vi "Controller Configuration Loop.vi"(7 "Sync Objects":T1, 8 "error in (no error)":errorcluster, 11 "FOFB Configuration":T5={"FOFB Parameters"={"Network"={"FOFB Controller IP"="", "LNLS Control Network IP"="", "LNLS Control Network Power Supplies TCP Port"=0, "LNLS Control Network FOFB Configuration TCP Port"=0, "Data Server TCP Port"=0, "Monitoring Data TCP Port"=0, "Configuration GUI TCP Port"=0, "TCP Listening Timeout"=0}, "Fast Acquisition"={"Acquisition Period"=0, "Data Buffer Size"=0}, "Response Matrix Measurement"={"Step Amplitude"=0.0, "Time Between Steps"=0, "Step Duration"=0, "Number of Averages"=0}, "Correction Algorithm"={"Correction Period"=0, "Reference Orbit Path"=path "", "Response Matrix Path"=path "", "Correction Matrix Path"=path "", "Horizontal Correction Factor"=0.0, "Vertical Correction Factor"=0.0, "Beam Current FOFB Threshold"=0.0, "Decouple H-V"=FALSE}, "Acquisition Network"=[], "Actuation Network"=[]}, "Number of Acquisition Chassis"=0, "Number of Actuation Chassis"=0, "Number of BPM Readings"=0, "BPM Reading Names"=[], "Selected BPM Readings"=[0, 1, 2, 3, 4, 5, 6, 7, 8, 9, 10, 11, 12, 13, 14, 15, 16, 17, 18, 19, 20, 21, 22, 23, 24, 25, 26, 27, 28, 29, 30, 31, 32, 33, 34, 35, 36, 37, 38, 39, 40, 41, 42, 43, 44, 45, 46, 47, 48, 49], "Number of Correctors"=0, "Corrector Names"=[], "Selected Correctors"=[0, 1, 2, 3, 4, 5, 6, 7, 8, 9, 10, 11, 12, 13, 14, 15, 16, 17, 18, 19, 20, 21, 22, 23, 24, 25, 26, 27, 28, 29, 30, 31, 32, 33, 34, 35, 36, 37, 38, 39, 40, 41, 42, 43, 44, 45, 46, 47, 48, 49], "Reference Orbit"=[], "Response Matrix"=[], "Correction Matrix"=[], "Acquisition Chassis Names"=[], "Actuation Chassis Names"=[], "Acquisition Variables"=[], "Actuation Variables"=[], "PS Matrix Mapping"=[], "Inverse PS Matrix Mapping"=[], "Response Matrix Beam Energy (MeV)"=0.0, "PID Parameters"=[], "BPM Planes"=[], "Corrector Planes"=[], "RMM Step Factor"=[]}) -> (0 "error out":errorcluster)   [LabVIEW 2011, in "Controller VIs.lvlib"]
uses:
  Controller VIs.lvlib
  Types Definitions/Type FOFB Configuration.ctl
  Types Definitions/Type FOFB Parameters.ctl
  Types Definitions/Type Network Configuration.ctl
  Types Definitions/Type FA Configuration.ctl
  Types Definitions/Type Response Matrix Measurement Configuration.ctl
  Types Definitions/Type Correction Algorithm Configuration.ctl
  Types Definitions/Type Acquisition Network Configuration.ctl
  Types Definitions/Type Actuation Network Configuration.ctl
  Types Definitions/Type PID Parameters.ctl
  Types Definitions/Type Synchronization Objects.ctl
  Types Definitions/Type Blocking Synchronization Objects.ctl
  Types Definitions/Type FA Request Parameters.ctl
  Types Definitions/Type BPM and PS select cluster.ctl
  Types Definitions/Type FA File Parameters.ctl
  Types Definitions/Type Monitoring Data.ctl
  Types Definitions/Type Diagnostics Data.ctl
  Types Definitions/Type CPU Loads Array.ctl
  Types Definitions/Type CPU Loads.ctl
  Types Definitions/Type Non-blocking Synchronization Objects.ctl
  Types Definitions/Type FOFB Variables.ctl
  Types Definitions/Type Actuation State.ctl
  <vilib>/Platform/TimedLoop/XDataNode/timing_clust.ctl
  <vilib>/Platform/TimedLoop/XDataNode/nitl_modes.ctl
  <vilib>/Platform/TimedLoop/XDataNode/wakeup.ctl
  Types Definitions/Type Configuration Data (GUI to Controller).ctl
  <vilib>/rtutility.llb/RT Debug String.vi
  <vilib>/Platform/TimedLoop/XDataNode/XDataNode.xnode
  Type Definitions.lvlib
  Log VIs.lvlib
  Misc VIs.lvlib
  <vilib>/Platform/TimedLoop/XDataNode/XDNodeRunTimeDep.lvlib
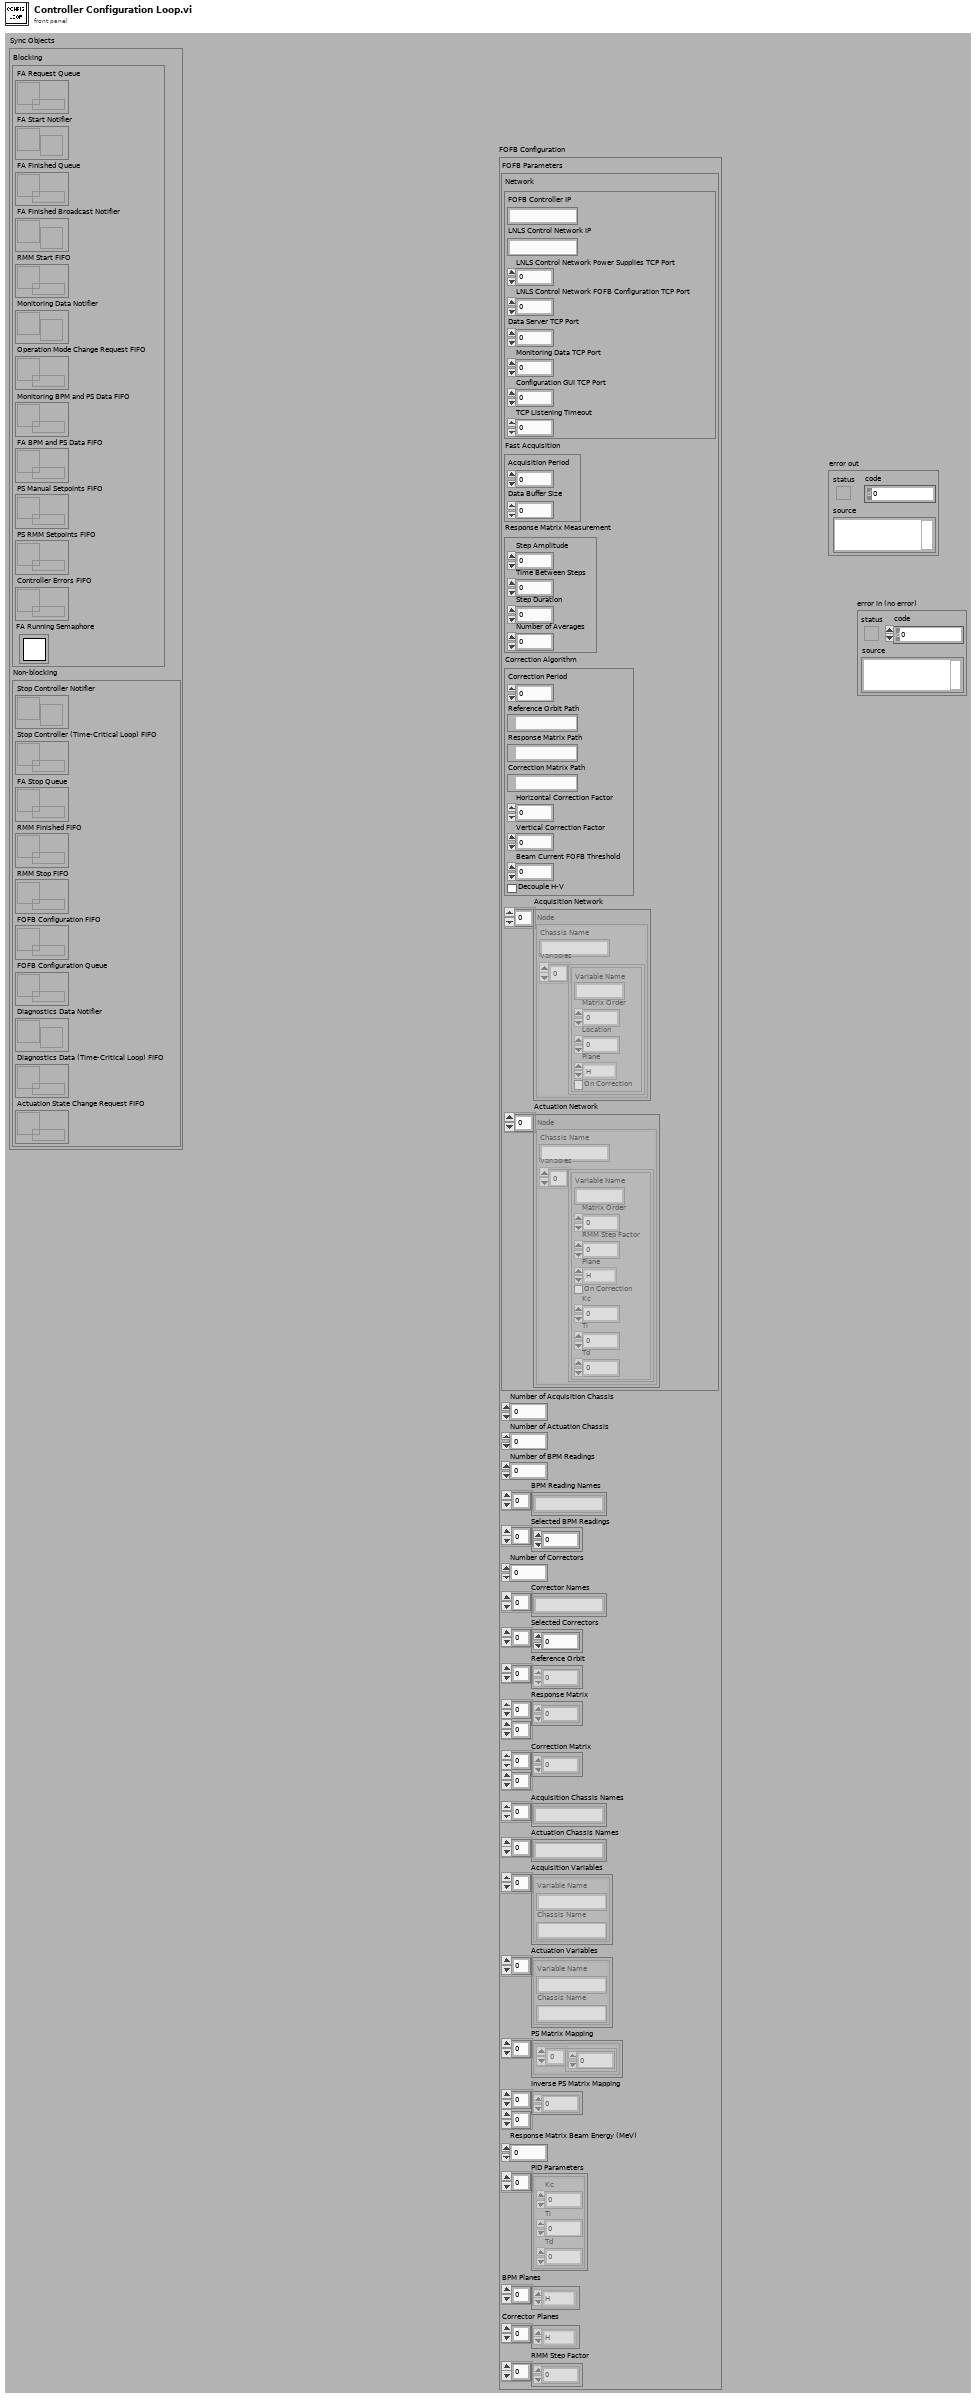
[diagram p1: front panel]
types:
  T1 = typedef "Type Definitions.lvlib/Type Synchronization Objects.ctl" = cluster{"Blocking":T2, "Non-blocking":T4}
  T2 = typedef "Type Definitions.lvlib/Type Blocking Synchronization Objects.ctl" = cluster{"FA Request Queue":refnum<queue>, "FA Start Notifier":refnum<notifier>, "FA Finished Queue":refnum<queue>, "FA Finished Broadcast Notifier":refnum<notifier>, "RMM Start FIFO":refnum<k33>, "Monitoring Data Notifier":refnum<notifier>, "Operation Mode Change Request FIFO":refnum<k33>, "Monitoring BPM and PS Data FIFO":refnum<k33>, "FA BPM and PS Data FIFO":refnum<k33>, "PS Manual Setpoints FIFO":refnum<k33>, "PS RMM Setpoints FIFO":refnum<k33>, "Controller Errors FIFO":refnum<k33>, "FA Running Semaphore":T3}
  T3 = typedef "Semaphore RefNum" = refnum<k1>
  T4 = typedef "Type Definitions.lvlib/Type Non-blocking Synchronization Objects.ctl" = cluster{"Stop Controller Notifier":refnum<notifier>, "Stop Controller (Time-Critical Loop) FIFO":refnum<k33>, "FA Stop Queue":refnum<queue>, "RMM Finished FIFO":refnum<k33>, "RMM Stop FIFO":refnum<k33>, "FOFB Configuration FIFO":refnum<k33>, "FOFB Configuration Queue":refnum<queue>, "Diagnostics Data Notifier":refnum<notifier>, "Diagnostics Data (Time-Critical Loop) FIFO":refnum<k33>, "Actuation State Change Request FIFO":refnum<k33>}
  T5 = typedef "Type Definitions.lvlib/Type FOFB Configuration.ctl" = cluster{"FOFB Parameters":T6, "Number of Acquisition Chassis":i32, "Number of Actuation Chassis":i32, "Number of BPM Readings":i32, "BPM Reading Names":string[], "Selected BPM Readings":u32[], "Number of Correctors":i32, "Corrector Names":string[], "Selected Correctors":u32[], "Reference Orbit":dbl[], "Response Matrix":dbl[][], "Correction Matrix":dbl[][], "Acquisition Chassis Names":string[], "Actuation Chassis Names":string[], "Acquisition Variables":cluster{"Variable Name":string, "Chassis Name":string}[], "Actuation Variables":cluster{"Variable Name":string, "Chassis Name":string}[], "PS Matrix Mapping":cluster{u32[]}[], "Inverse PS Matrix Mapping":u32[][], "Response Matrix Beam Energy (MeV)":dbl, "PID Parameters":T13[], "BPM Planes":enum8{"H", "V"}[], "Corrector Planes":enum8{"H", "V"}[], "RMM Step Factor":dbl[]}
  T6 = typedef "Type Definitions.lvlib/Type FOFB Parameters.ctl" = cluster{"Network":T7, "Fast Acquisition":T8, "Response Matrix Measurement":T9, "Correction Algorithm":T10, "Acquisition Network":T11, "Actuation Network":T12}
  T7 = typedef "Type Definitions.lvlib/Type Network Configuration.ctl" = cluster{"FOFB Controller IP":string, "LNLS Control Network IP":string, "LNLS Control Network Power Supplies TCP Port":u16, "LNLS Control Network FOFB Configuration TCP Port":u16, "Data Server TCP Port":u16, "Monitoring Data TCP Port":u16, "Configuration GUI TCP Port":u16, "TCP Listening Timeout":i32}
  T8 = typedef "Type Definitions.lvlib/Type FA Configuration.ctl" = cluster{"Acquisition Period":u32, "Data Buffer Size":u32}
  T9 = typedef "Type Definitions.lvlib/Type Response Matrix Measurement Configuration.ctl" = cluster{"Step Amplitude":dbl, "Time Between Steps":u32, "Step Duration":u32, "Number of Averages":u32}
  T10 = typedef "Type Definitions.lvlib/Type Correction Algorithm Configuration.ctl" = cluster{"Correction Period":u32, "Reference Orbit Path":path, "Response Matrix Path":path, "Correction Matrix Path":path, "Horizontal Correction Factor":dbl, "Vertical Correction Factor":dbl, "Beam Current FOFB Threshold":dbl, "Decouple H-V":bool}
  T11 = typedef "Type Definitions.lvlib/Type Acquisition Network Configuration.ctl" = cluster{"Chassis Name":string, "Variables":cluster{"Variable Name":string, "Matrix Order":u32, "Location":dbl, "Plane":enum8{"H", "V"}, "On Correction":bool}[]}[]
  T12 = typedef "Type Definitions.lvlib/Type Actuation Network Configuration.ctl" = cluster{"Chassis Name":string, "Variables":cluster{"Variable Name":string, "Matrix Order":u32, "RMM Step Factor":dbl, "Plane":enum8{"H", "V"}, "On Correction":bool, "Kc":dbl, "Ti":dbl, "Td":dbl}[]}[]
  T13 = typedef "Type Definitions.lvlib/Type PID Parameters.ctl" = cluster{"Kc":fxp<+/-,16,8>, "Ti":fxp<+/-,16,8>, "Td":fxp<+/-,16,8>}
  T14 = enum16{"Idle", "Wait Connection", "Read Data", "Process Data", "Write Data", "Close Connection"}
  T15 = typedef "XDNodeRunTimeDep.lvlib/timing_clust.ctl" = cluster{"Expected End [f-1]":u64, "Actual End [f-1]":u64, "Finished Late? [f-1]":bool, "Expected End [i-1]":u64, "Actual End [i-1]":u64, "Finished Late? [i-1]":bool, "Expected Start [i]":u64, "Actual Start [i]":u64, "Expected Start [f]":u64, "Actual Start [f]":u64, "Source Name":string, "Structure Name":string, "Period":i64, "Deadline":i64, "Offset":i64, "Start":i64, "Priority":i32, "Timeout":i32, "Mode":T16, "Wakeup Reason":T17, "Error":errorcluster, "Source Type":string, "Secondary Source Type":string, "Global End Time":u64, "Global Start Time":u64, "Frame Duration":u64, "Iteration Duration":u64, "Assigned CPU":i32, "I/O Scan Engine Mode":u32}
  T16 = typedef "XDNodeRunTimeDep.lvlib/nitl_modes.ctl" = enum32{"No Change", "Process missed periods, maintain original phase", "Discard missed periods, maintain original phase", "Process missed periods, ignore original phase", "Discard missed periods, ignore original phase"}
  T17 = typedef "XDNodeRunTimeDep.lvlib/wakeup.ctl" = enum32{"Normal", "Aborted", "Asynchronous wakeup", "Timing source error", "Timed loop error", "Timeout"}
  T18 = typedef "Type Definitions.lvlib/Type Configuration Data (GUI to Controller).ctl" = cluster{"Operation Mode":enum16{"Idle Mode", "Error Mode", "Manual Mode", "FOFB Mode", "RMM Mode"}[], "Update Controller Soft Configuration":bool[], "Trigger RT Execution Trace":string[]}
  T19 = typedef "Type Definitions.lvlib/Type Configuration Change Acknowledge (Controller to GUI).ctl" = cluster{"Operation Mode ACK":bool[]}
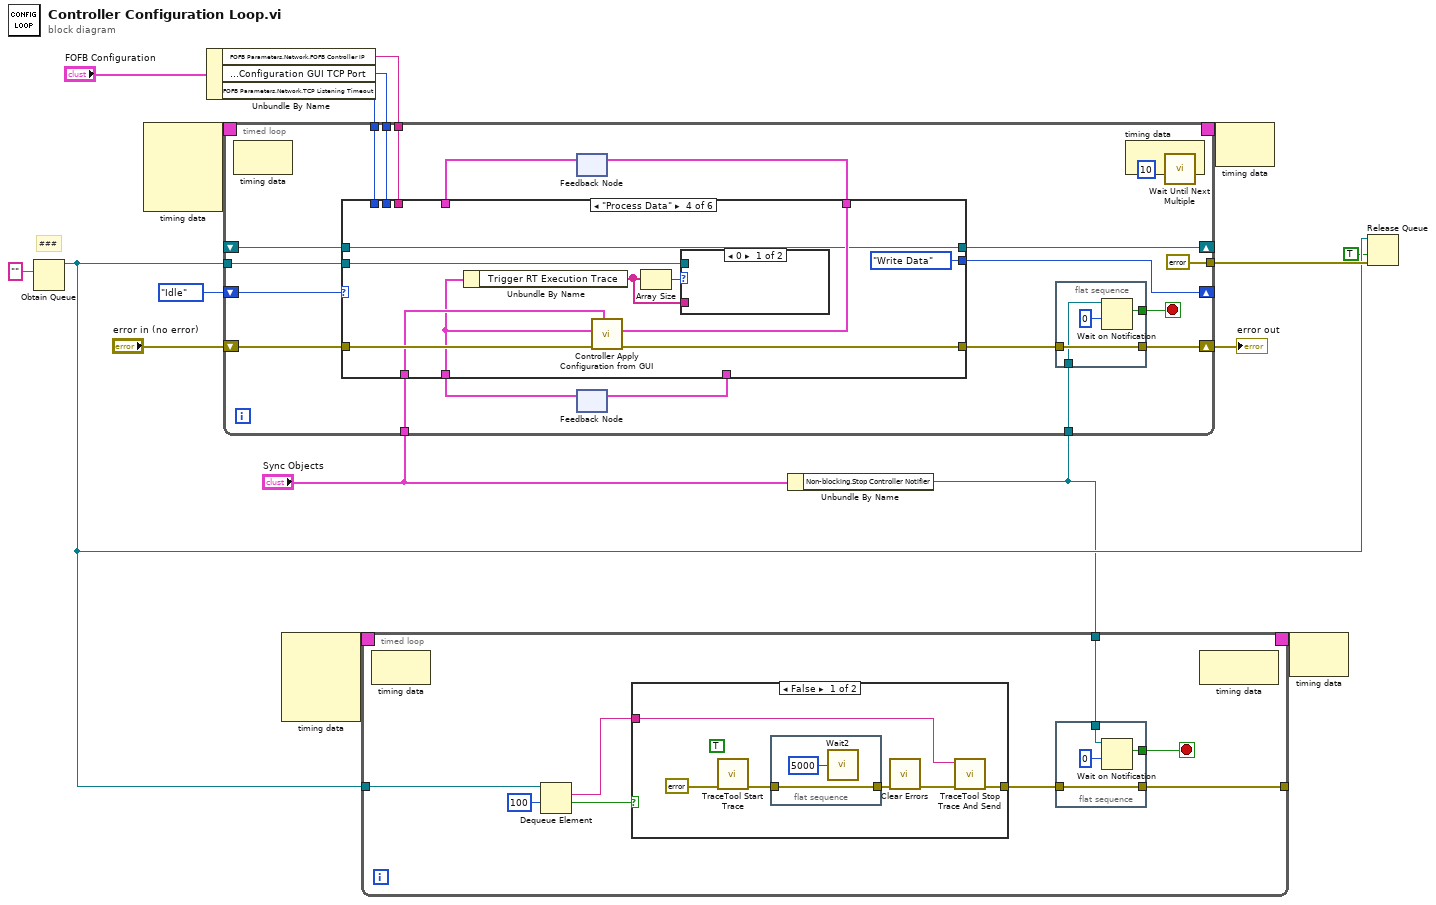
[diagram p0: block diagram]
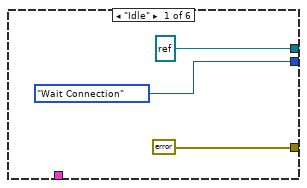
[diagram p3: hidden frame]
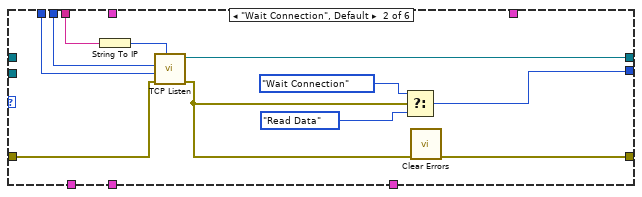
[diagram p4: hidden frame]
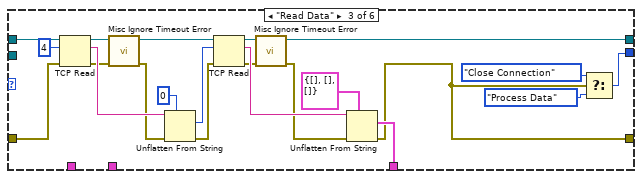
[diagram p5: hidden frame]
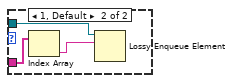
[diagram p6: hidden frame]
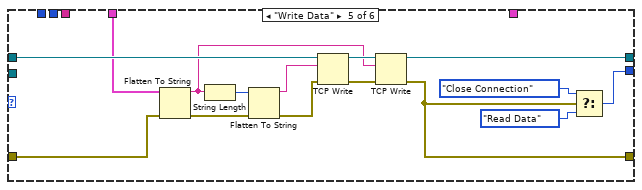
[diagram p7: hidden frame]
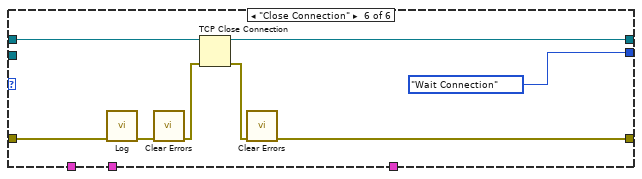
[diagram p8: hidden frame]
diagram:
  # "###"
  n1 = Obtain Queue(element data type="" ("Host IP Address")) -> (queue out=w3:refnum<queue>)  [unwired: 4 in, 2 out]
  n2 = node-c288() -> (w9:T15)  [unwired: 4 in]
  n3 = Unbundle By Name("FOFB Configuration") -> ("FOFB Parameters.Network.FOFB Controller IP"=w16:string, "FOFB Parameters.Network.Configuration GUI TCP Port"=w10:u16, "FOFB Parameters.Network.TCP Listening Timeout"=w15:i32)
  n4 = node-c288() -> (w7:T15)  [unwired: 4 in]
  n5 = Unbundle By Name("Sync Objects") -> ("Non-blocking.Stop Controller Notifier"=w1:refnum<notifier>)
  n6 = timed-loop {
    tunnel: w16 -> [w37]
    tunnel: w10 -> [w36]
    tunnel: w15 -> [w35]
    shift-right: [w23] -> w13
    shift-left: "error in (no error)" -> [w32]
    shift-right: [w30] -> _
    shift-left: T14."Idle" ("f") -> [w31]
    shift-right: [w33] -> _
    shift-left: _ -> [w34]
    tunnel: w1 -> [w22]
    tunnel: "Sync Objects" -> [w27]
    timing: w9 -> [_]
    timing-out: [_] -> w8
    tunnel: w3 -> [w19]
    tunnel: [errorcluster {"status"=FALSE, "code"=0, "source"=""} ("error out")] -> w4
    stop <- w21 stop-if-true
    # "ms"
    n7 = node-c288() -> ()  [unwired: 1 in, 1 out]
    n8 = feedback #1() -> (w26:T19)  [unwired: 1 in]
    n9 = feedback #2() -> (w28:T18)  [unwired: 1 in]
    n10 = case shown="\"Process Data\"" w31 {
      tunnel: [refnum<k5> refnum ("connection ID") w57 w70 w84 w105 w113] -> w33
      tunnel: [T14."Wait Connection" ("f") w56 w66 T14."Write Data" ("f") w104 T14."Wait Connection" ("f")] -> w30
      tunnel: [errorcluster {"status"=FALSE, "code"=0, "source"=""} ("error out") w54 w58 w86 w103 w112] -> w24
      tunnel: w32 -> [_ w53 w69 w87 w93 w107]
      tunnel: w34 -> [_ _ w71 w84 w101 w106]
      tunnel: w37 -> [_ w52 _ _ _ _]
      tunnel: w36 -> [_ w50 _ _ _ _]
      tunnel: w35 -> [_ w49 _ _ _ _]
      tunnel: [_ _ w63 _ _ _] -> w29
      tunnel: w28 -> [_ _ _ w81 _ _]
      tunnel: w27 -> [_ _ _ w82 _ _]
      tunnel: w26 -> [_ _ _ _ w94 _]
      tunnel: [_ _ _ w85 _ _] -> w25
      tunnel: w19 -> [_ _ _ w78 _ _]
      frame "Idle" {
      }
      frame "Wait Connection", Default {
        n11 = String To IP(1:w52) -> (0:w51:u32)
        n12 = call <vilib>:"TCP Listen.vi"("net address"=w51, "error in (no error)"=w53, "timeout ms (wait forever: -1)"=w49, "port"=w50) -> ("error out"=w55:errorcluster, "connection ID"=w57:refnum<k5>)  [unwired: 3 in, 3 out]
        n13 = Select(t=T14."Wait Connection" ("f"), s=w55, f=T14."Read Data") -> (s? t:f=w56:T14)
        n14 = call <vilib>:"Clear Errors.vi"("error in (no error)"=w55) -> ("error out"=w54:errorcluster)  [unwired: 6 out]
      }
      frame "Read Data" {
        n15 = TCP Read(connection ID=w71, bytes to read=4, error in (no error)=w69) -> (connection ID out=w77:refnum<k5>, data out=w75:string, error out=w64:errorcluster)  [unwired: 2 in]
        n16 = call "Misc Ignore Timeout Error.vi"("error in (no error)"=w64) -> ("error out"=w62:errorcluster)  [unwired: 10 in]
        n17 = Unflatten From String(type=0 ("bytes to read"), binary string=w75, error in (no error)=w62) -> (value=w73:i32, error out=w61:errorcluster)  [unwired: 2 in, 1 out]
        n18 = TCP Read(connection ID=w77, bytes to read=w73, error in (no error)=w61) -> (connection ID out=w70:refnum<k5>, data out=w72:string, error out=w60:errorcluster)  [unwired: 2 in]
        n19 = call "Misc Ignore Timeout Error.vi"("error in (no error)"=w60) -> ("error out"=w59:errorcluster)  [unwired: 10 in]
        n20 = Unflatten From String(type=T18 {"Operation Mode"=[], "Update Controller Soft Configuration"=[], "Trigger RT Execution Trace"=[]} ("Configuration Data (GUI to Controller)"), binary string=w72, error in (no error)=w59) -> (value=w63:T18, error out=w58:errorcluster)  [unwired: 2 in, 1 out]
        n21 = Select(t=T14."Close Connection" ("f"), s=w58, f=T14."Process Data") -> (s? t:f=w66:T14)
      }
      frame "Process Data" {
        n22 = Unbundle By Name(w81) -> ("Trigger RT Execution Trace"=w79:string[])
        n23 = call "Controller Apply Configuration from GUI.vi"("Sync Objects"=w82, "error in (no error)"=w87, "Configuration Data (GUI to Controller)"=w81) -> ("error out"=w86:errorcluster, "Configuration Change Acknowledge (Controller to GUI)"=w85:T19)  [unwired: 7 in]
        n24 = Array Size(array=w79) -> (size(s)=w80:i32)
        n25 = case shown="0" w80 {
          tunnel: w79 -> [_ w90]
          tunnel: w78 -> [_ w88]
          frame 0 {
          }
          frame 1, Default {
            n26 = Index Array(array=w90) -> (element=w89:string)  [unwired: 1 in]
            n27 = Lossy Enqueue Element(queue=w88, element=w89) -> ()  [unwired: 1 in, 4 out]
          }
        }
      }
      frame "Write Data" {
        n28 = Flatten To String(anything=w94, error in (no error)=w93) -> (data string=w97:string, error out=w92:errorcluster)  [unwired: 2 in, 1 out]
        n29 = String Length(string=w97) -> (length=w99:i32)
        n30 = Flatten To String(anything=w99, error in (no error)=w92) -> (data string=w98:string, error out=w91:errorcluster)  [unwired: 2 in, 1 out]
        n31 = TCP Write(connection ID=w101, data in=w98, error in (no error)=w91) -> (connection ID out=w102:refnum<k5>, error out=w100:errorcluster)  [unwired: 2 out]
        n32 = TCP Write(connection ID=w102, data in=w97, error in (no error)=w100) -> (connection ID out=w105:refnum<k5>, error out=w103:errorcluster)  [unwired: 2 out]
        n33 = Select(t=T14."Close Connection" ("f"), s=w103, f=T14."Read Data") -> (s? t:f=w104:T14)
      }
      frame "Close Connection" {
        n34 = call "Log.vi"("error in (no error)"=w107) -> ("error out"=w110:errorcluster)  [unwired: 9 in, 1 out]
        n35 = call <vilib>:"Clear Errors.vi"("error in (no error)"=w110) -> ("error out"=w111:errorcluster)  [unwired: 6 in]
        n36 = TCP Close Connection(connection ID=w106, error in (no error)=w111) -> (connection ID out=w113:refnum<k5>, error out=w109:errorcluster)  [unwired: 1 in]
        n37 = call <vilib>:"Clear Errors.vi"("error in (no error)"=w109) -> ("error out"=w112:errorcluster)  [unwired: 6 in]
      }
    }
    n38 = feedback-in #1(w25) -> ()
    n39 = feedback-in #2(w29) -> ()
    n40 = flat-sequence {
      tunnel: [w42] -> w21
      tunnel: w24 -> [w41]
      tunnel: [w41] -> w23
      tunnel: w22 -> [w40]
      frame #0 {
        n41 = Wait on Notification(notifier=w40, timeout in ms (-1)=0) -> (notification=w42:bool)  [unwired: 2 in, 3 out]
      }
    }
    n42 = node-c288() -> ()  [unwired: 1 in, 1 out]
    n43 = call "Wait Until Next Multiple"("Count(mSec)"=u32 10) -> ()  [unwired: 1 out]
  }
  "error out" <- w13
  n44 = timed-loop {
    timing: w7 -> [_]
    timing-out: [_] -> w6
    tunnel: w3 -> [w119]
    tunnel: [w117] -> _
    tunnel: w1 -> [w116]
    stop <- w114 stop-if-true
    n45 = node-c288() -> ()  [unwired: 1 in, 1 out]
    n46 = Dequeue Element(queue=w119, timeout in ms (-1)=100) -> (element=w115:string, timed out?=w120:bool)  [unwired: 1 in, 2 out]
    n47 = case shown="False" w120 {
      tunnel: [w127 _] -> w118
      tunnel: w115 -> [w126 _]
      frame False {
        (unwired) TRUE ("Detailed Tracing? (F)")
        n48 = call <vilib>:"TraceTool Start Trace.vi"("error in (no error)"=errorcluster {"status"=FALSE, "code"=0, "source"=""} ("error out")) -> ("error out"=w130:errorcluster)  [unwired: 9 in, 1 out]
        n49 = flat-sequence {
          tunnel: w130 -> [w132]
          tunnel: [w132] -> w129
          frame #0 {
            n50 = call "Wait2"("Count(mSec)"=u32 5000) -> ()  [unwired: 1 out]
          }
        }
        n51 = call <vilib>:"Clear Errors.vi"("error in (no error)"=w129) -> ("error out"=w131:errorcluster)  [unwired: 6 in]
        n52 = call <vilib>:"TraceTool Stop Trace And Send.vi"("error in (no error)"=w131, "Trace Host Network Address"=w126) -> ("error out"=w127:errorcluster)  [unwired: 9 in]
      }
      frame True {
      }
    }
    n53 = flat-sequence {
      tunnel: [w124] -> w114
      tunnel: w118 -> [w123]
      tunnel: [w123] -> w117
      tunnel: w116 -> [w122]
      frame #0 {
        n54 = Wait on Notification(notifier=w122, timeout in ms (-1)=0) -> (notification=w124:bool)  [unwired: 2 in, 3 out]
      }
    }
    n55 = node-c288() -> ()  [unwired: 1 in, 1 out]
  }
  n56 = node-c288(w8) -> ()  [unwired: 1 out]
  n57 = node-c288(w6) -> ()  [unwired: 1 out]
  n58 = Release Queue(queue=w3, force destroy? (F)=TRUE, error in (no error)=w4) -> ()  [unwired: 3 out]
